vi "Build Delete.vi"(8 "error in (no error)":errorcluster, 9 "tableName":string, 10 "DynamicParameters in":refnum<class "DynamicParameters.lvclass">, 11 "KDBConnection in":refnum<class "DBC.lvclass">) -> (0 "error out":errorcluster, 2 "Query":string, 3 "KDBConnection out":refnum<class "DBC.lvclass">)   [LabVIEW 2020, in "ORM_DBC_Kdb.lvlib" / "DBC.lvclass"]
uses:
  DBC.lvclass
  C:/Program Files/National Instruments/LabVIEW 2020/vi.lib/Viviota/shared/ORM.lvlibp/ORM/DbConnection/DbConnection.lvclass
  <vilib>/Viviota/shared/ORM.lvlibp/ORM/DynamicParameters/DynamicParameters.lvclass
  <vilib>/Viviota/shared/ORM.lvlibp/ORM/DbConnection/Read ColumnNameEqualsValueFormat.vi
  <vilib>/Viviota/shared/ORM.lvlibp/ORM/DbConnection/Write ExecuteScalar.vi
  <vilib>/Viviota/shared/ORM.lvlibp/ORM/DynamicParameters/Read FieldNames.vi
  <vilib>/Viviota/shared/ORM.lvlibp/ORM/DynamicParameters/Read ParameterNames.vi
  <vilib>/Viviota/shared/ORM.lvlibp/ORM/DynamicParameters/Read ParameterOptions.vi
  <vilib>/Viviota/shared/ORM.lvlibp/ORM/DynamicParameters/Read AutoKey.vi
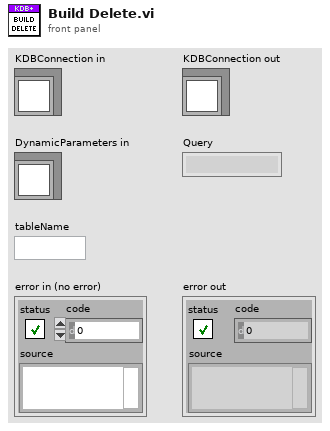
[diagram p1: front panel]
types:
  T1 = cluster{"DbType":i32, "Direction":i32, "Size":i32, "Precision":u8, "Scale":u8}[]
  T2 = typedef "ORM_DBC_Kdb.lvlib/DBC.lvclass/kdb_TableType_enum.ctl" = enum16{"Memory", "Disk_Serialized", "Disk_Splayed", "Disk_Partitioned", "Other"}
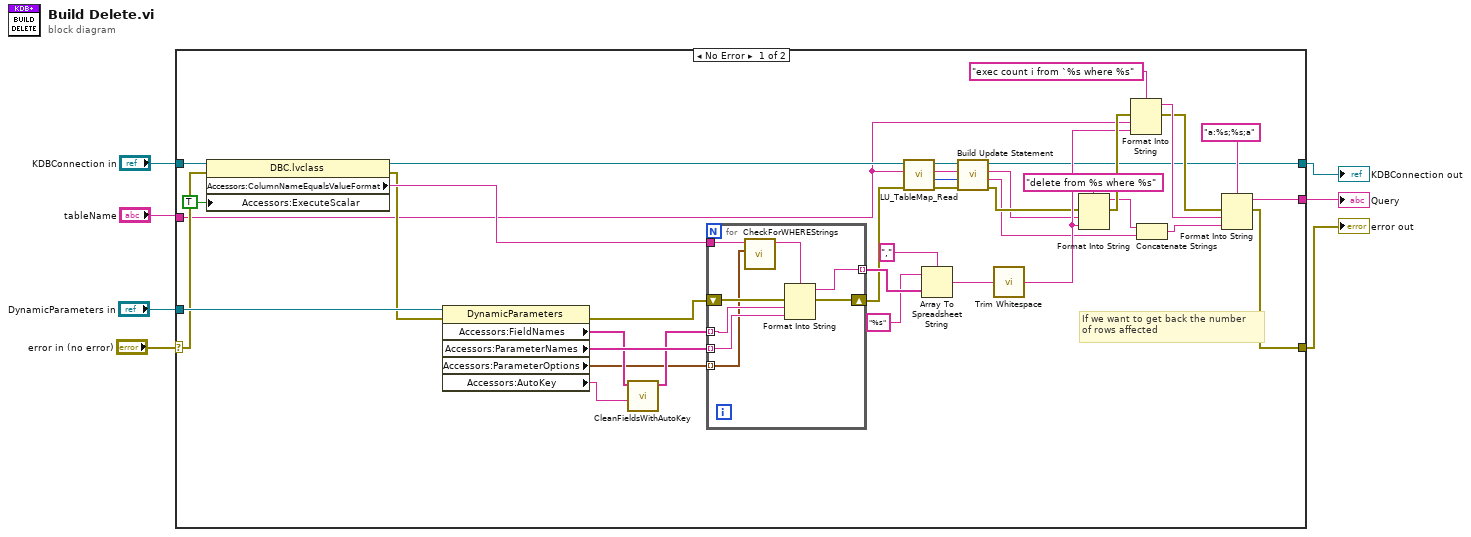
[diagram p0: block diagram]
diagram:
  n1 = case shown="No Error" "error in (no error)" {
    selector: "error in (no error)" -> [w40 w55]
    tunnel: [w27 w55] -> w1
    tunnel: [w15 w54] -> w3
    tunnel: "KDBConnection in" -> [w45 w54]
    tunnel: "DynamicParameters in" -> [w44 _]
    tunnel: "tableName" -> [w14 _]
    tunnel: [w32 _] -> w2
    frame No Error {
      # "If we want to get back the number\nof rows affected"
      n2 = property class="DBC.lvclass"(reference=w45, error in=w40, "Accessors:ExecuteScalar"=TRUE ("ExecuteScalar")) -> (reference out=w16:refnum<class "DBC.lvclass">, error out=w39:errorcluster, "Accessors:ColumnNameEqualsValueFormat"=w42:string)
      n3 = property class="DynamicParameters"(reference=w44, error in=w39) -> (error out=w38:errorcluster, "Accessors:FieldNames"=w23:string[], "Accessors:ParameterNames"=w43:string[], "Accessors:ParameterOptions"=w21:T1, "Accessors:AutoKey"=w25:string)  [unwired: 1 out]
      n4 = call "CleanFieldsWithAutoKey.vi"("AutoKey"=w25, "FieldNames"=w23) -> ("FieldNames_Clean"=w24:string[])  [unwired: 8 in, 1 out]
      n5 = for {
        tunnel: w24 -> [w50] mode=indexing
        tunnel: w43 -> [w51] mode=indexing
        tunnel: w42 -> [w48]
        tunnel: [w52] -> w41 mode=indexing
        shift-right: [w49] -> w13
        shift-left: w38 -> [w53]
        tunnel: w21 -> [w46] mode=indexing
        n6 = call "CheckForWHEREStrings.vi"("Options"=w46, "ColumnNameEqualsValueFormat in"=w48) -> ("ColumnNameEqualsValueFormat out"=w47:string)  [unwired: 9 in]
        n7 = Format Into String(format string=w47, error in=w53, w50, w51) -> (resulting string=w52:string, error out=w49:errorcluster)  [unwired: 1 in]
      }
      n8 = call "LU_TableMap_Read.vi"("error in (no error)"=w13, "TableName"=w14, "KDBConnection in"=w16) -> ("error out"=w19:errorcluster, "TableType"=w17:T2, "TableName Out"=w18:string, "KDBConnection out"=w20:refnum<class "DBC.lvclass">)  [unwired: 5 in]
      n9 = Array To Spreadsheet String(delimiter (Tab)=",", array=w41, 3:"%s" ("format string")) -> (spreadsheet string=w35:string)
      n10 = call "Build Update Statement.vi"("error in (no error)"=w19, "TableType"=w17, "TableName Out"=w18, "KDBConnection in"=w20) -> ("error out"=w12:errorcluster, "Update Suffix Command"=w8:string, "Table to Use"=w11:string, "KDBConnection out"=w15:refnum<class "DBC.lvclass">)  [unwired: 4 in]
      n11 = call <vilib>:"Trim Whitespace.vi"("string"=w35) -> ("trimmed string"=w22:string)  [unwired: 1 in]
      n12 = Format Into String(format string="delete from %s where %s", error in=w12, w11, w22) -> (resulting string=w10:string, error out=w29:errorcluster)  [unwired: 1 in]
      n13 = Format Into String(format string="exec count i from `%s where %s", error in=w29, w14, w22) -> (resulting string=w30:string, error out=w28:errorcluster)  [unwired: 1 in]
      n14 = Concatenate Strings(w10, w8) -> (w9:string)
      n15 = Format Into String(format string="a:%s;%s;a", error in=w28, w30, w9) -> (resulting string=w32:string, error out=w27:errorcluster)  [unwired: 1 in]
    }
    frame Error {
    }
  }
  "error out" <- w1
  "KDBConnection out" <- w3
  "Query" <- w2
